vi "circuits-capacitor.vi"(1 "Invert Y":bool, 2 "Invert X":bool, 4 "L2":dbl=0.05, 5 "L3":dbl=0.5, 6 "Swap-XY":bool, 7 "L1":dbl=0.1, 8 "Device in Y":refnum<k24>, 9 "GetPOS Y":refnum<vi>, 10 "GetPOS X":refnum<vi>, 11 "Device in X":refnum<k24>) -> (0 "Device out Y":refnum<k24>, 3 "Device out X":refnum<k24>)   [LabVIEW 2014]
doc: "André Romero - 2019\nandretec@ifsc.usp.br"
uses:
  C:/users-lab/Andre/GITs/andretec/Thorlabs-Vector-Move/kinesisTec/Kinesis/Thorlabs.MotionControl.TCube.DCServoCLI.dll
  Kinesis/Thorlabs.MotionControl.TCube.DCServoCLI.dll
panel:
  out "-x":dbl=-0.5
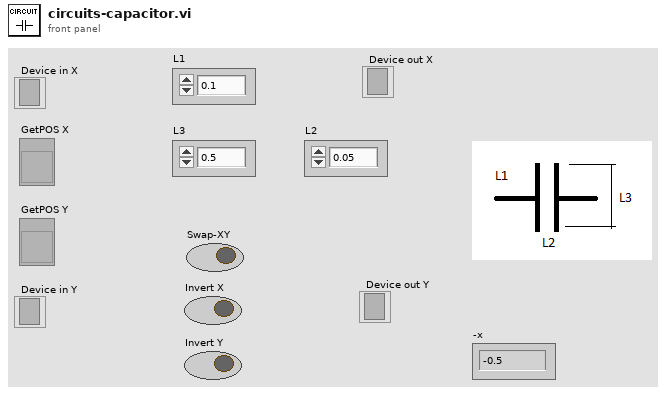
[diagram p1: front panel]
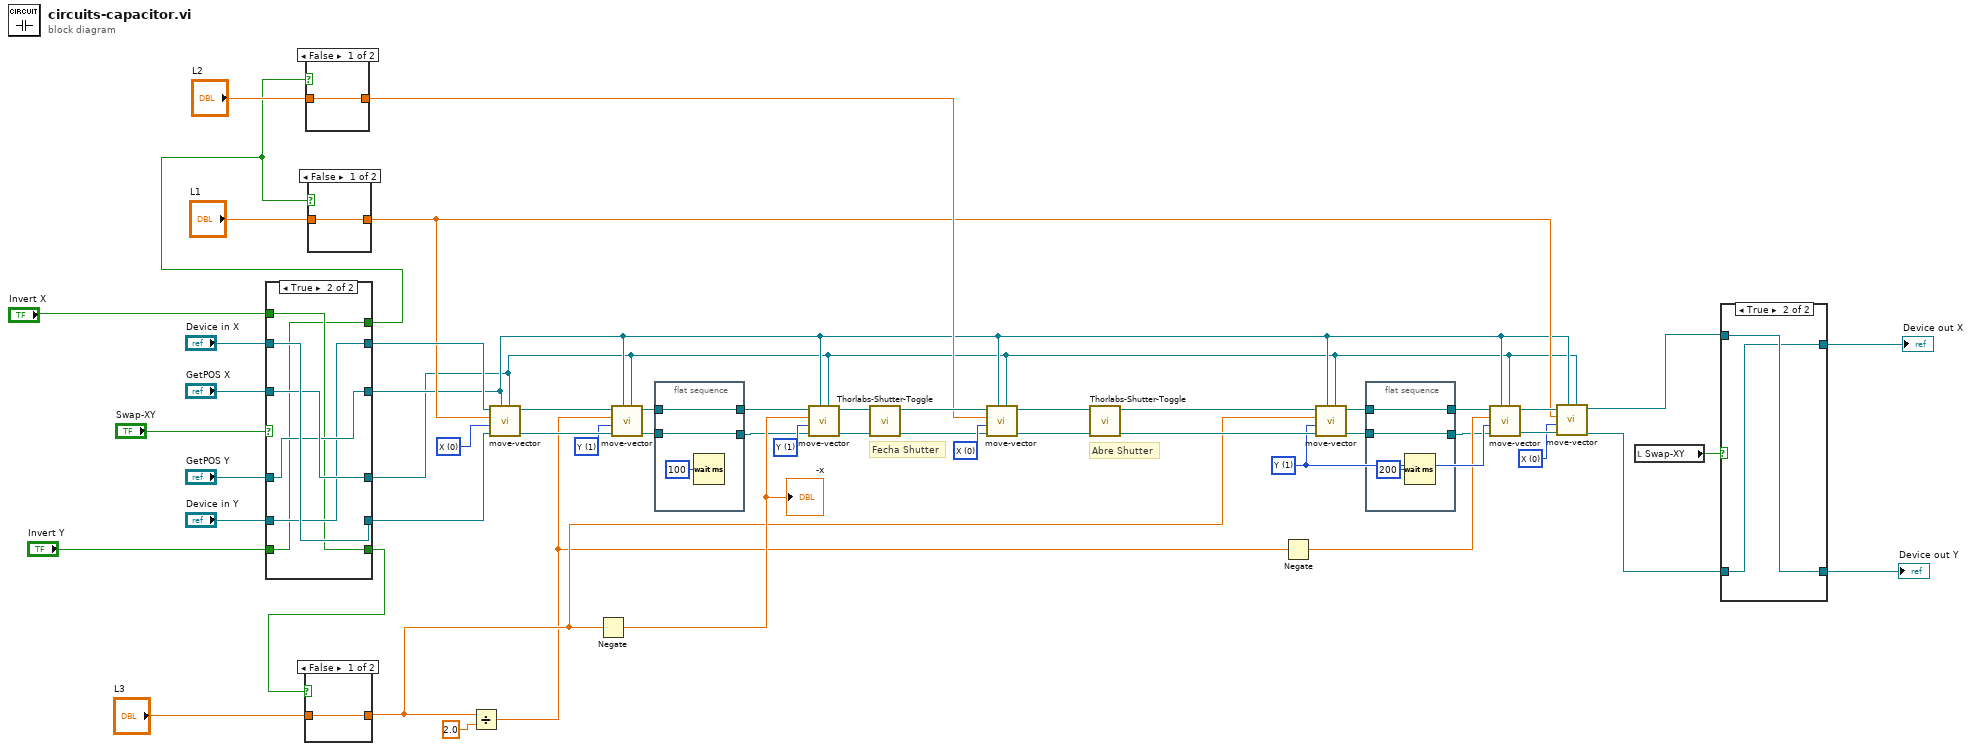
[diagram p0: block diagram]
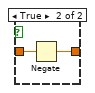
[diagram p3: hidden frame]
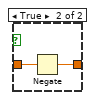
[diagram p4: hidden frame]
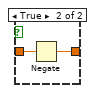
[diagram p5: hidden frame]
diagram:
  w18 = u16 1 items=["X", "Y"] ("X-Y")
  w21 = u16 0 items=["X", "Y"] ("X-Y")
  w27 = u16 1 items=["X", "Y"] ("X-Y")
  w41 = u16 0 items=["X", "Y"] ("X-Y")
  w35 = u16 1 items=["X", "Y"] ("X-Y")
  w45 = u16 0 items=["X", "Y"] ("X-Y")
  # "Abre Shutter"
  # "Fecha Shutter"
  n1 = case shown="True" "Swap-XY" {
    tunnel: "Device in X" -> [w58 w66]
    tunnel: [w58 w63] -> w47
    tunnel: "GetPOS Y" -> [w60 w64]
    tunnel: [w60 w65] -> w19
    tunnel: "Device in Y" -> [w59 w63]
    tunnel: [w59 w66] -> w46
    tunnel: "GetPOS X" -> [w57 w65]
    tunnel: [w57 w64] -> w20
    tunnel: "Invert X" -> [w56 w62]
    tunnel: [w56 w61] -> w8
    tunnel: "Invert Y" -> [w55 w61]
    tunnel: [w55 w62] -> w6
    frame False {
    }
    frame True {
    }
  }
  n2 = case shown="False" w6 {
    tunnel: "L3" -> [w67 w69]
    tunnel: [w67 w68] -> w28
    frame False {
    }
    frame True {
      n3 = Negate(x=w69) -> (-x=w68:dbl)
    }
  }
  n4 = case shown="False" w8 {
    tunnel: "L2" -> [w70 w72]
    tunnel: [w70 w71] -> w29
    frame False {
    }
    frame True {
      n5 = Negate(x=w72) -> (-x=w71:dbl)
    }
  }
  n6 = case shown="False" w8 {
    tunnel: "L1" -> [w73 w75]
    tunnel: [w73 w74] -> w22
    frame False {
    }
    frame True {
      n7 = Negate(x=w75) -> (-x=w74:dbl)
    }
  }
  n8 = Divide(x=w28, y=2.0) -> (x/y=w26:dbl)
  n9 = call "move-vector.vi"("GetPOS Y"=w19, "GetPOS X"=w20, "Device in Y"=w46, "X-Y"=w45, "Distance"=w22, "Device in X"=w47) -> ("Device out Y"=w43:refnum<k24>, "Device out X"=w44:refnum<k24>)  [unwired: 4 in]
  n10 = Negate(x=w28) -> (-x=w32:dbl)
  "-x" <- w32
  n11 = call "move-vector.vi"("GetPOS Y"=w19, "GetPOS X"=w20, "Device in Y"=w43, "X-Y"=w35, "Distance"=w26, "Device in X"=w44) -> ("Device out Y"=w15:refnum<k24>, "Device out X"=w17:refnum<k24>)  [unwired: 4 in]
  n12 = flat-sequence {
    tunnel: [w78] -> w16
    tunnel: w17 -> [w78]
    tunnel: w15 -> [w77]
    tunnel: [w77] -> w14
    frame #0 {
      n13 = Wait (ms)(milliseconds to wait=u32 100) -> ()  [unwired: 1 out]
    }
  }
  n14 = call "move-vector.vi"("GetPOS Y"=w19, "GetPOS X"=w20, "Device in Y"=w14, "X-Y"=w18, "Distance"=w32, "Device in X"=w16) -> ("Device out Y"=w33:refnum<k24>, "Device out X"=w34:refnum<k24>)  [unwired: 4 in]
  n15 = call "Thorlabs-Shutter-Toggle.vi"("Device in Y"=w33, "Device in X"=w34) -> ("Device out Y"=w40:refnum<k24>, "Device out X"=w42:refnum<k24>)  [unwired: 8 in]
  n16 = call "move-vector.vi"("GetPOS Y"=w19, "GetPOS X"=w20, "Device in Y"=w40, "X-Y"=w41, "Distance"=w29, "Device in X"=w42) -> ("Device out Y"=w38:refnum<k24>, "Device out X"=w39:refnum<k24>)  [unwired: 4 in]
  n17 = call "Thorlabs-Shutter-Toggle.vi"("Device in Y"=w38, "Device in X"=w39) -> ("Device out Y"=w36:refnum<k24>, "Device out X"=w37:refnum<k24>)  [unwired: 8 in]
  n18 = Negate(x=w26) -> (-x=w25:dbl)
  n19 = call "move-vector.vi"("GetPOS Y"=w19, "GetPOS X"=w20, "Device in Y"=w36, "X-Y"=w27, "Distance"=w28, "Device in X"=w37) -> ("Device out Y"=w12:refnum<k24>, "Device out X"=w13:refnum<k24>)  [unwired: 4 in]
  n20 = flat-sequence {
    tunnel: [w81] -> w11
    tunnel: w13 -> [w81]
    tunnel: w12 -> [w80]
    tunnel: [w80] -> w10
    frame #0 {
      n21 = Wait (ms)(milliseconds to wait=u32 200) -> ()  [unwired: 1 out]
    }
  }
  n22 = call "move-vector.vi"("GetPOS Y"=w19, "GetPOS X"=w20, "Device in Y"=w10, "X-Y"=w27, "Distance"=w25, "Device in X"=w11) -> ("Device out Y"=w23:refnum<k24>, "Device out X"=w24:refnum<k24>)  [unwired: 4 in]
  n23 = call "move-vector.vi"("GetPOS Y"=w19, "GetPOS X"=w20, "Device in Y"=w23, "X-Y"=w21, "Distance"=w22, "Device in X"=w24) -> ("Device out Y"=w3:refnum<k24>, "Device out X"=w4:refnum<k24>)  [unwired: 4 in]
  n24 = local read "Swap-XY"() -> (w5:bool)
  n25 = case shown="True" w5 {
    tunnel: w4 -> [w83 w85]
    tunnel: [w83 w84] -> w2
    tunnel: w3 -> [w82 w84]
    tunnel: [w82 w85] -> w1
    frame False {
    }
    frame True {
    }
  }
  "Device out X" <- w2
  "Device out Y" <- w1
